vi "GetNodeCall.vi"(5 "name":string, 6 "error in":errorcluster, 9 "PythonConverter_BD in":refnum<class "PyConvBD.lvclass">) -> (0 "error out":errorcluster, 3 "PythonConverter_BD out":refnum<class "PyConvBD.lvclass">, 4 "call":T1)   [LabVIEW 2014, in "Raspberry Pi Compatible Compiler for LabVIEW.lvlib" / "PyConvBD.lvclass"]
uses:
  PyConvBD.lvclass
  TypeDefs/NodeCall_TD.ctl
  PyConvBD.lvclass/PyConvBD.ctl
  Raspberry Pi Compatible Compiler for LabVIEW.lvlib
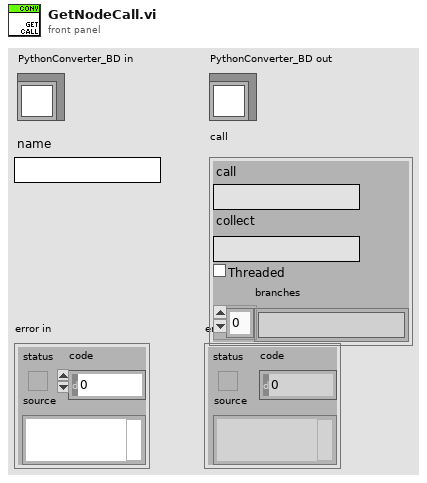
[diagram p1: front panel]
types:
  T1 = typedef "Raspberry Pi Compatible Compiler for LabVIEW.lvlib/NodeCall_TD.ctl" = cluster{"call":string, "collect":string, "Threaded":bool, "branches":string[]}
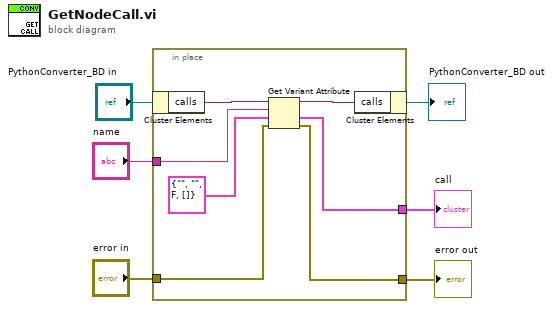
[diagram p0: block diagram]
diagram:
  n1 = in-place {
    in-place-border: "error in" -> [w12]
    in-place-border: [w11] -> w3
    in-place-border: "name" -> [w10]
    in-place-border: [w8] -> w1
    n2 = in-place-cluster #1("PythonConverter_BD in") -> ("calls"=w9:variant)
    n3 = Get Variant Attribute(Variant=w9, name=w10, default value (empty Variant)=T1 {"call"="", "collect"="", "Threaded"=FALSE, "branches"=[]} ("call"), error in=w12) -> (duplicate Variant=w13:variant, value=w8:T1, error out=w11:errorcluster)  [unwired: 1 out]
    n4 = in-place-cluster #1("calls"=w13) -> (→"PythonConverter_BD out":refnum<class "PyConvBD.lvclass">)
  }
  "error out" <- w3
  "call" <- w1
